vi "init_web_polling.vi"(8 "error in (no error)":errorcluster, 10 "base path":path, 11 "simple_html_chat_ui in":refnum<class "simple_html_chat_ui.lvclass">) -> (0 "error out":errorcluster, 3 "simple_html_chat_ui out":refnum<class "simple_html_chat_ui.lvclass">)   [LabVIEW 2020, in "simple_html_chat_ui.lvclass"]
doc: "To run the web polling VI"
uses:
  simple_html_chat_ui.lvclass
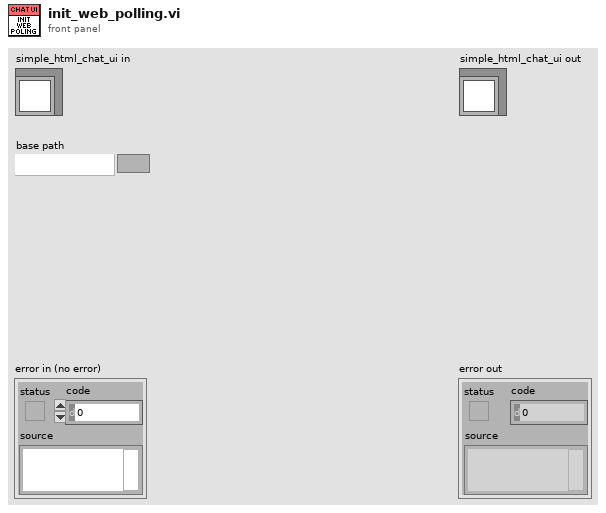
[diagram p1: front panel]
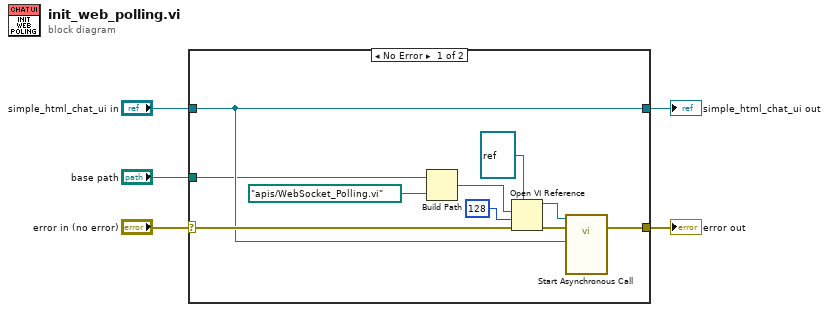
[diagram p0: block diagram]
diagram:
  n1 = case shown="No Error" "error in (no error)" {
    selector: "error in (no error)" -> [w8 w17]
    tunnel: [w9 w17] -> w4
    tunnel: [w7 w16] -> w2
    tunnel: "simple_html_chat_ui in" -> [w7 w16]
    tunnel: "base path" -> [w6 _]
    frame No Error {
      n2 = Build Path(base path=w6, name or relative path=path "apis/WebSocket_Polling.vi") -> (appended path=w12:path)
      n3 = Open VI Reference(type specifier VI Refnum (for type only)=refnum<vi> refnum, vi path=w12, options=128, error in (no error)=w8) -> (vi reference=w13:refnum<vi>, error out=w14:errorcluster)  [unwired: 2 in]
      n4 = call-by-ref "Start Asynchronous Call"(reference=w13, error in=w14, "simple_html_chat_ui in"=w7) -> (error out=w9:errorcluster)  [unwired: 9 in, 3 out]
    }
    frame Error {
    }
  }
  "error out" <- w4
  "simple_html_chat_ui out" <- w2
